vi "Get Current Log File Instance.vi"(8 "error in (no error)":errorcluster, 11 "Segmented Log in":refnum<class "Segmented Log.lvclass">) -> (0 "error out":errorcluster, 2 "Log File Instance":refnum<class "Log File.lvclass">, 3 "Segmented Log out":refnum<class "Segmented Log.lvclass">)   [LabVIEW 2015, in "Segmented Log.lvclass"]
uses:
  Segmented Log.lvclass
  Log Files/Log File/Log File.lvclass
  Segmented Log.lvclass/Segmented Log.ctl
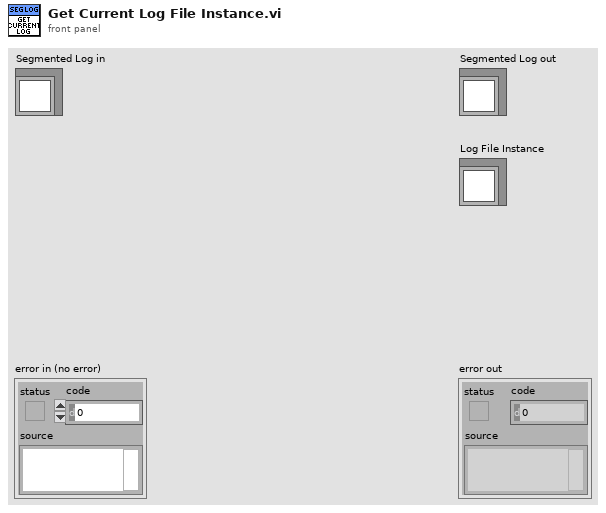
[diagram p1: front panel]
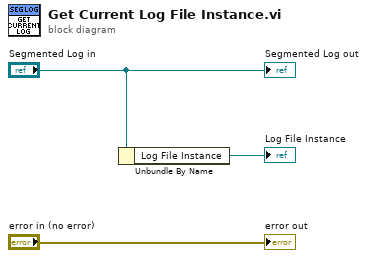
[diagram p0: block diagram]
diagram:
  n1 = Unbundle By Name("Segmented Log in") -> ("Log File Instance"=→"Log File Instance":refnum<class "Log File.lvclass">)
  "error out" <- "error in (no error)"
  "Segmented Log out" <- "Segmented Log in"
